vi "Measurement UI.vi"() -> ()   [LabVIEW 2023, in "Crosstalk_Class D Amplifier UI.lvlib"]
uses:
  Crosstalk_Class D Amplifier UI.lvlib
  shared/controls/digital output level units.ctl
  shared/ui/controls/view.ctl
  UI State.ctl
  <vilib>/Utility/miscctls.llb/LVBoundsTypeDef.ctl
  <vilib>/Utility/miscctls.llb/LVPoint32TypeDef.ctl
  <vilib>/Utility/miscctls.llb/LVPointTypeDef.ctl
  shared/ui/UI Helpers.lvlib
  shared/audio popup ui/Audio Popup UI.lvlib
  shared/controls/audio controls.lvlib
panel:
  in  "view legend":T1
  out "time domain":waveform(dbl)[](graph)
  out "frequency domain":T2(graph)
  out "meas table":string[][](table)
  in  "digital serial cfg file":string
  out "output power (W)":dbl[](array[numeric])
  out "crosstalk (dB)":dbl[](array[numeric])
  out "frequency (Hz)":dbl[](array[numeric])
  out "channel names":string[](array[string])
  in  "acq channel - interferer":string caption="Interferrer channel resource"
  in  "acq channel - victim":string caption="Victim channel resource"
  out "wfm_interferrer - data":dbl[](array[numeric])
  out "fft_interferrer - data":dbl[](array[numeric])
  in  "Configuration tab":enum32{"Protocol", "Measurement"}(tab)
  out "digital serial file name":string
  in  "configure digital serial":bool
  in  "master clock channel list":string caption="Master Clock Channel"
  in  "digital channel list":string caption="Digital Audio Channel"
  in  "Interferer channel resource":tag
  in  "Victim channel resource":tag
  in  "output level":dbl=-1.0 caption="Output level" format="%#_3f"
  in  "output level units":T3=enum."dBFS"
  in  "min settling cycles":u32 caption="Minimum settling cycles"
  in  "min settling time (s)":dbl=0.1 caption="Minimum settling time" format="%#_6ps"
  in  "min measurement cycles":u32 caption="Minimum measurement cycles"
  in  "min measurement time (s)":dbl=0.1 caption="Minimum measurement time" format="%#_6ps"
  in  "lowpass filter":T4(ring) caption="Lowpass filter"
  in  "highpass filter":enum32{"DC", "AC"}(ring) caption="Highpass filter"
  in  "load impedance":dbl=-1.0 caption="Load impedance" format="%#_6p Ohms"
  in  "digital audio interferer channel":i32 caption="Interferer channel"
  in  "output range (pk-pk)":dbl=15.0 caption="Output range" format="%.3p Vpk-pk"
  in  "signal frequency":dbl=1000.0 caption="Frequency" format="%#_6pHz"
  in  "acq sampling rate":dbl=51200.0 caption="Sample rate" format="%#.6pHz"
  in  "channel 0 offset":u32=1
  out "fft_victim - data":dbl[](array[numeric])
  out "fft - df":dbl
  out "fft - f0":dbl
  out "wfm_victim - data":dbl[](array[numeric])
  out "wfm - dt":dbl
  in  "acq channel":string="PXI1Slot4/ai0"
  in  "signal phase":dbl caption="phase"
  # "hidden controls - used to sync with MeasLink"
  # "hidden indicators"
  # "Digital Serial Settings"
  # "Harware Resource"
  # "Filters"
  # "Output"
  # "Acquisition"
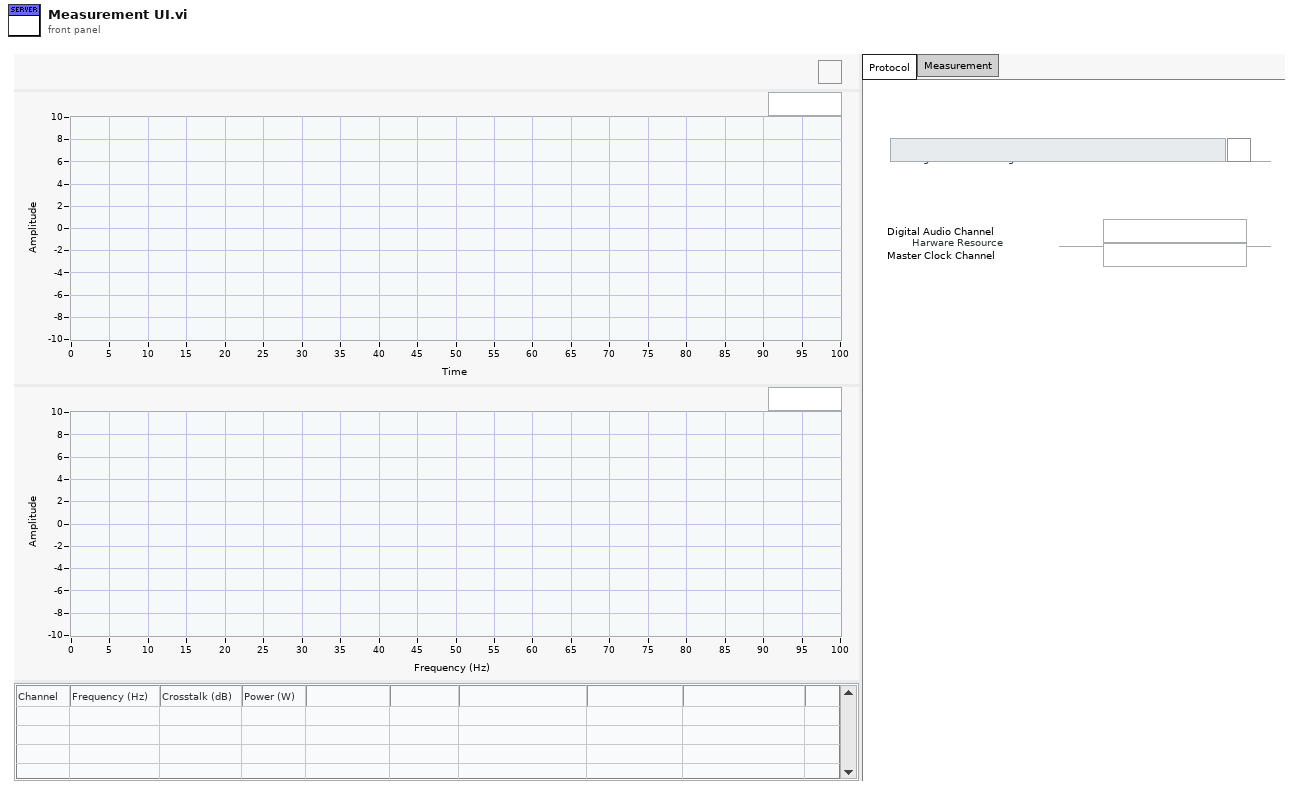
[diagram p1: front panel]
types:
  T1 = typedef "UI Helpers.lvlib/view.ctl" = bool
  T2 = cluster{"fft - f0":dbl, "fft - df":dbl, "fft_interferrer - data":dbl[]}[]
  T3 = typedef "audio controls.lvlib/digital output level units.ctl" = enum32{"% FS", "dBFS", "V"}
  T4 = enum32{"No filter", "AES17 20kHz", "AES17 40kHz"}
  T5 = typedef "Crosstalk_Class D Amplifier UI.lvlib/UI State.ctl" = cluster{"Graph Size":T6, "Legend Visible":bool, "Mouse Coords":T7, "PostUI event occurred":bool, "digital serial cfg file":path}
  T6 = typedef "LVBoundsTypeDef.ctl" = cluster{"Width":u32, "Height":u32}
  T7 = typedef "LVPoint32TypeDef.ctl" = cluster{"Horizontal":i32, "Vertical":i32}
  T8 = typedef "LVPointTypeDef.ctl" = cluster{"Horizontal":i16, "Vertical":i16}
  T9 = typedef "Audio Popup UI.lvlib/audio settings.ctl" = cluster{"digital serial file":string}
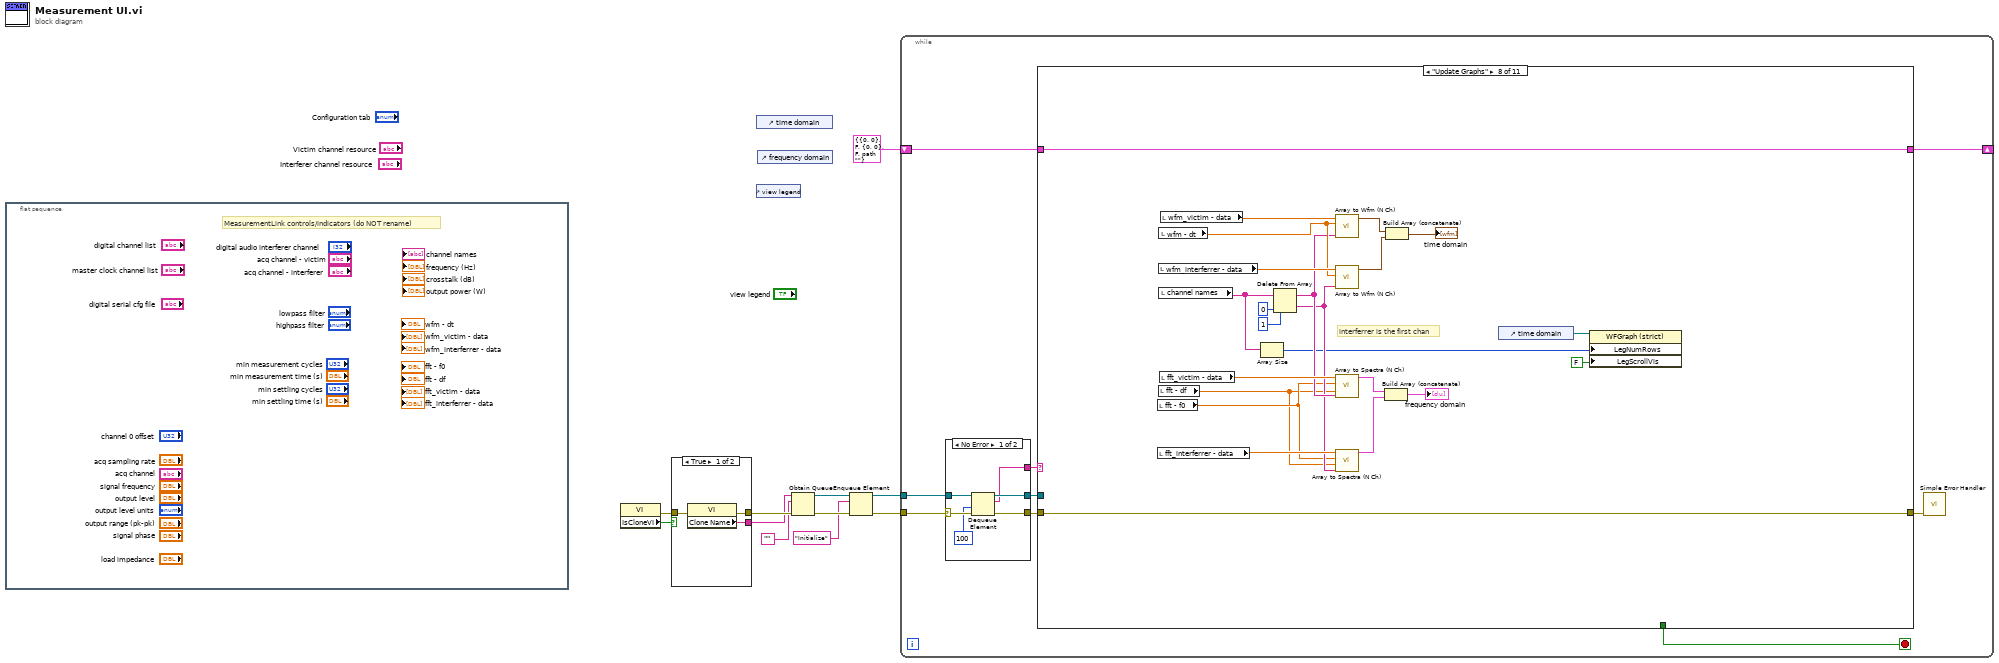
[diagram p0: block diagram]
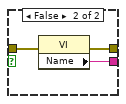
[diagram p2: hidden frame]
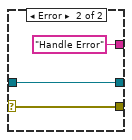
[diagram p3: hidden frame]
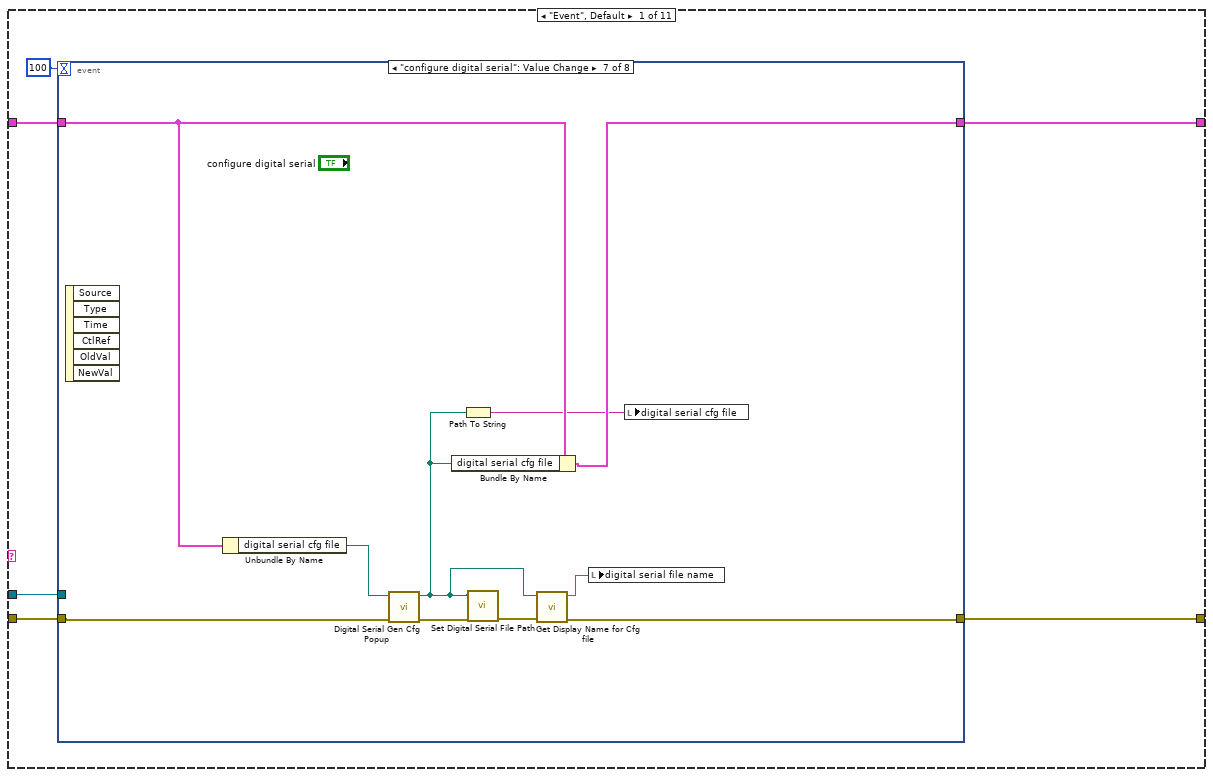
[diagram p4: hidden frame]
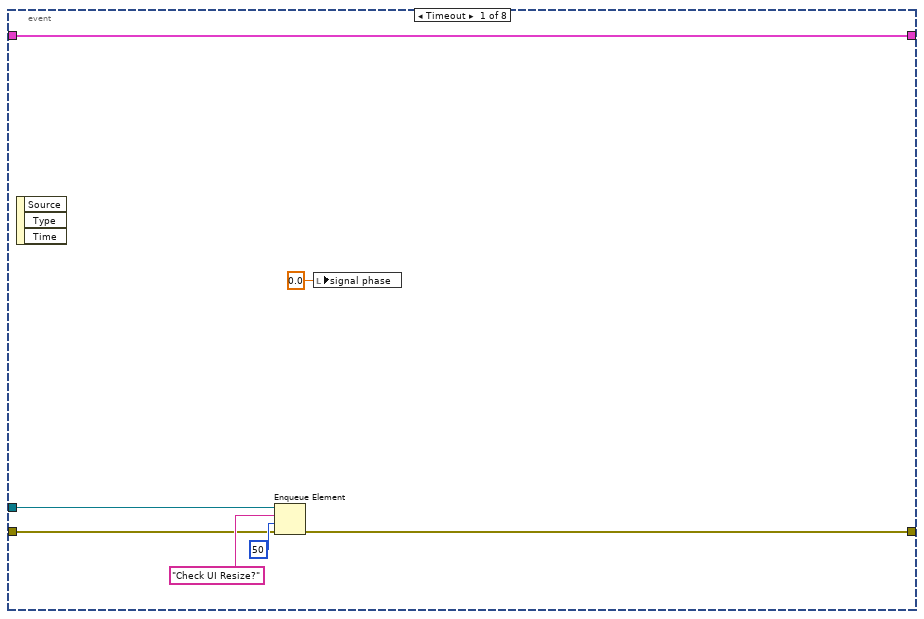
[diagram p5: hidden frame]
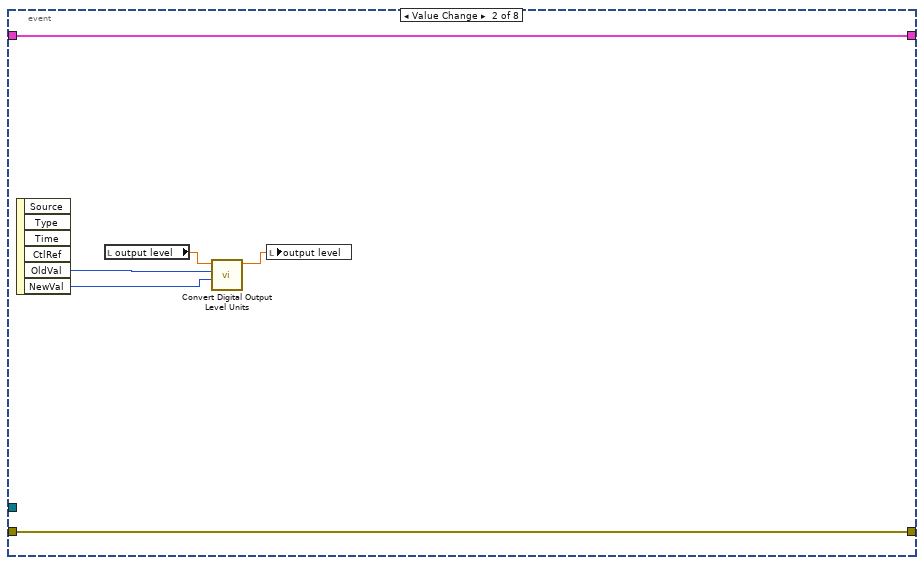
[diagram p6: hidden frame]
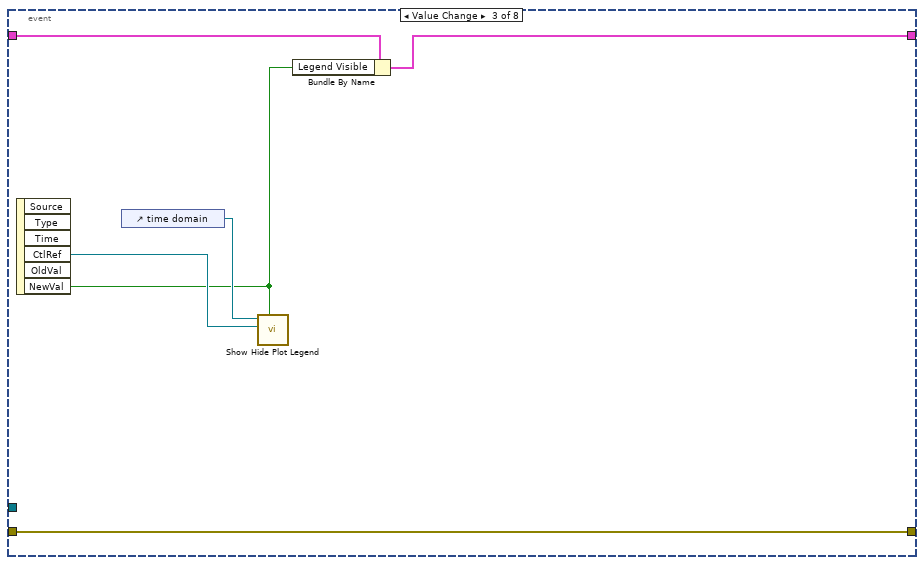
[diagram p7: hidden frame]
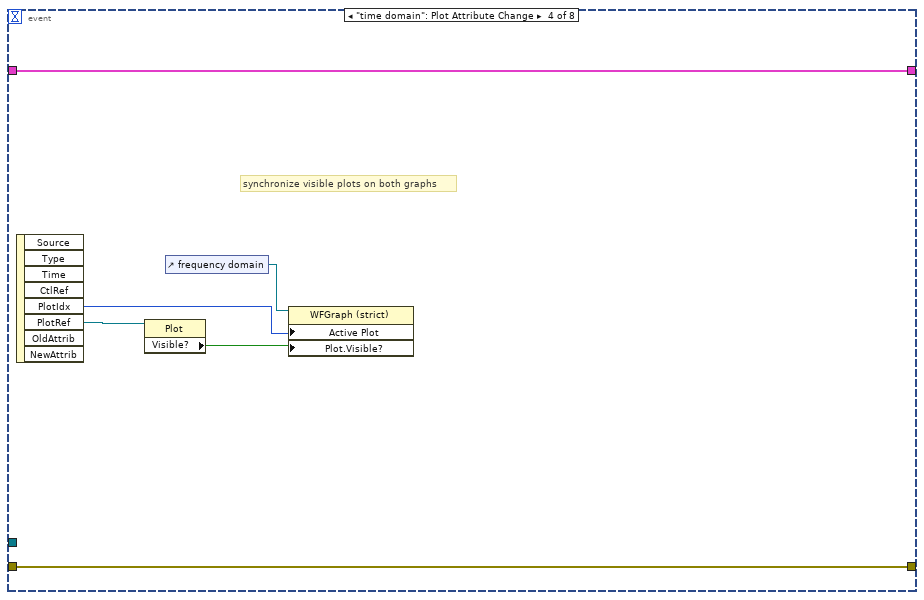
[diagram p8: hidden frame]
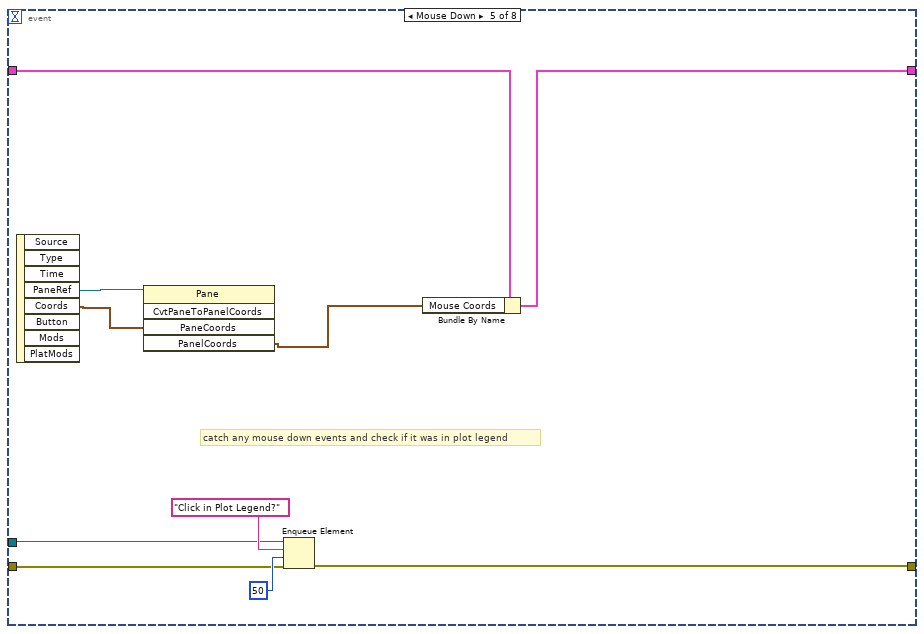
[diagram p9: hidden frame]
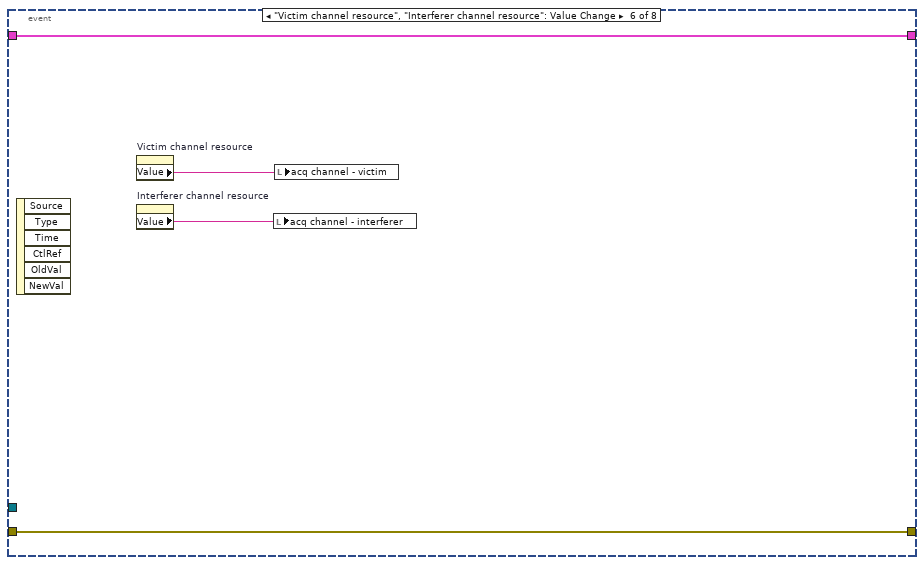
[diagram p10: hidden frame]
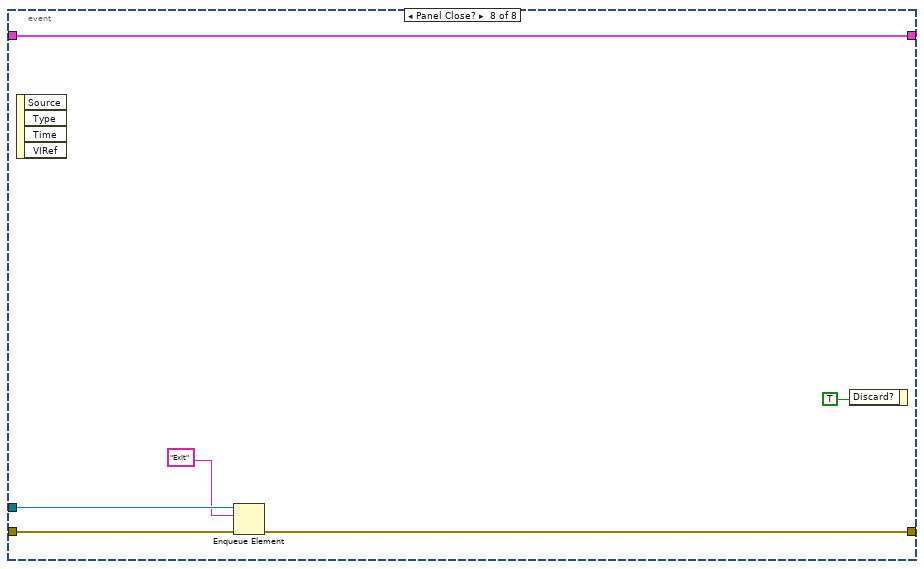
[diagram p11: hidden frame]
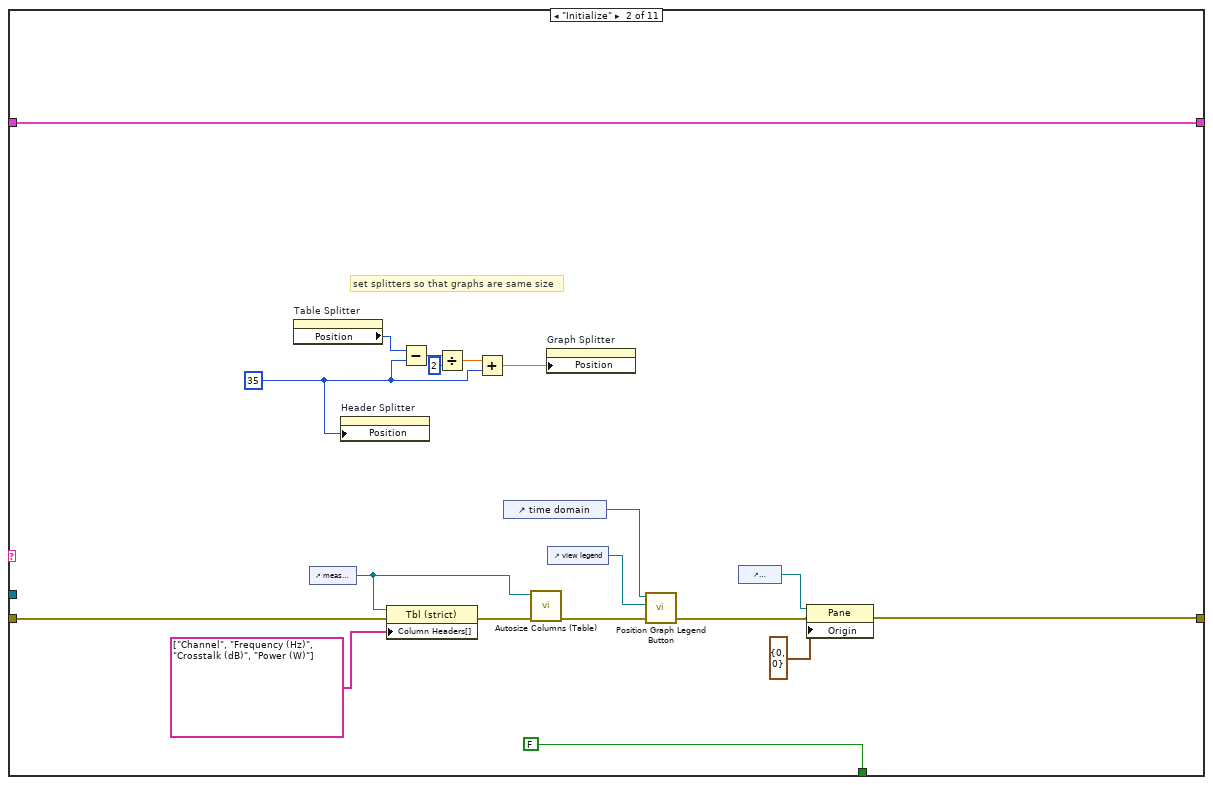
[diagram p12: hidden frame]
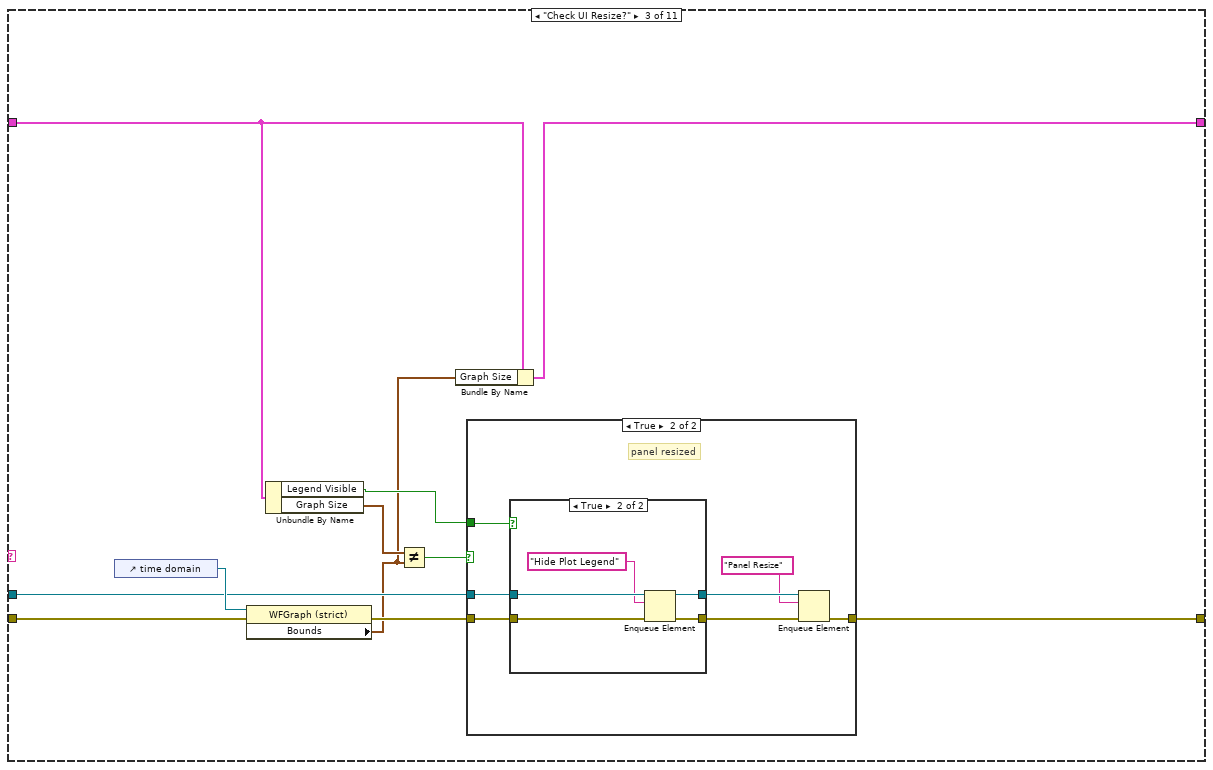
[diagram p13: hidden frame]
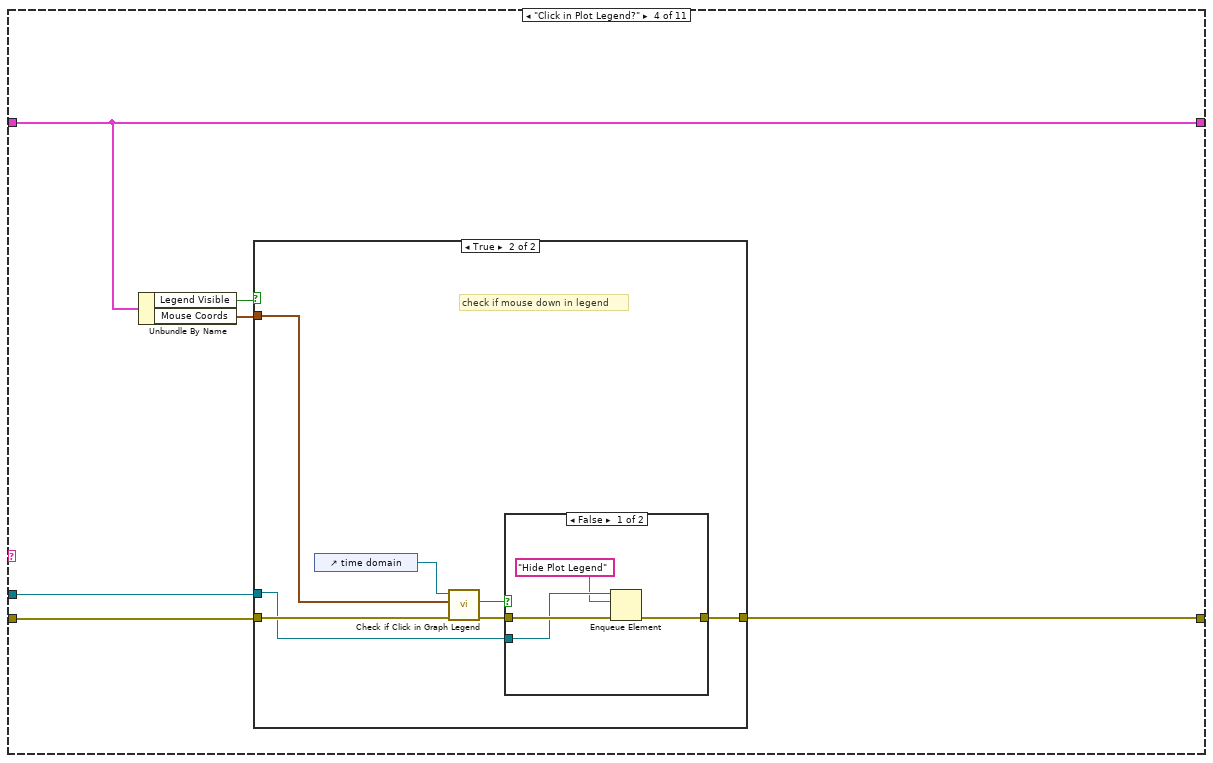
[diagram p16: hidden frame]
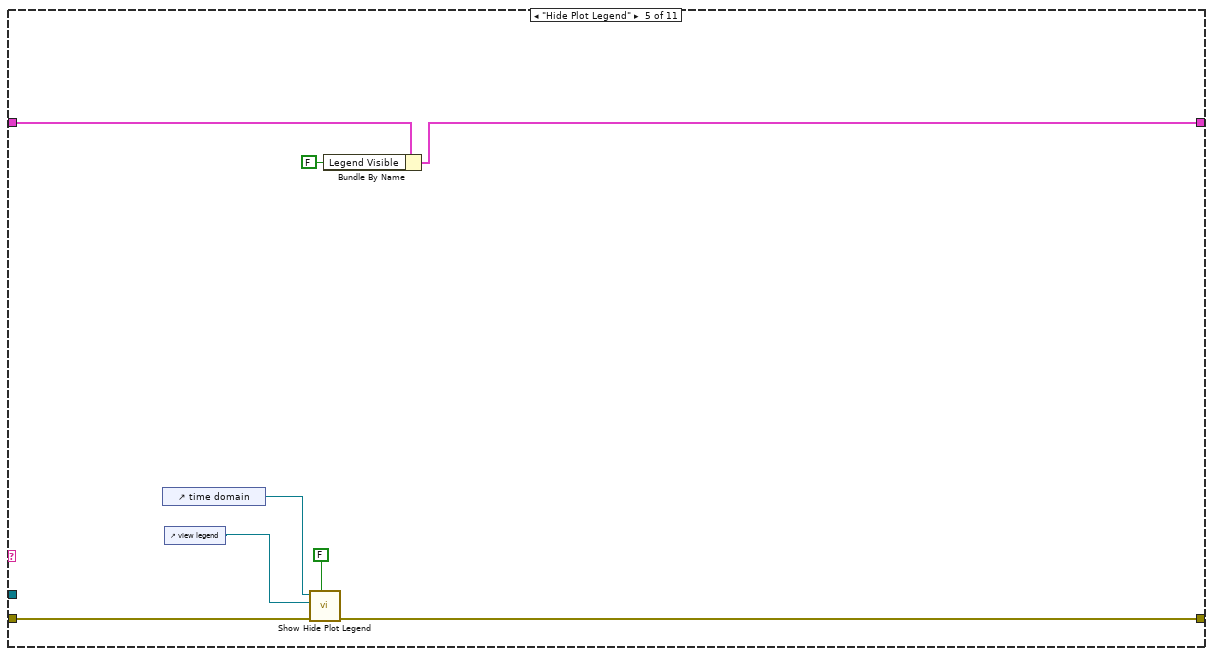
[diagram p19: hidden frame]
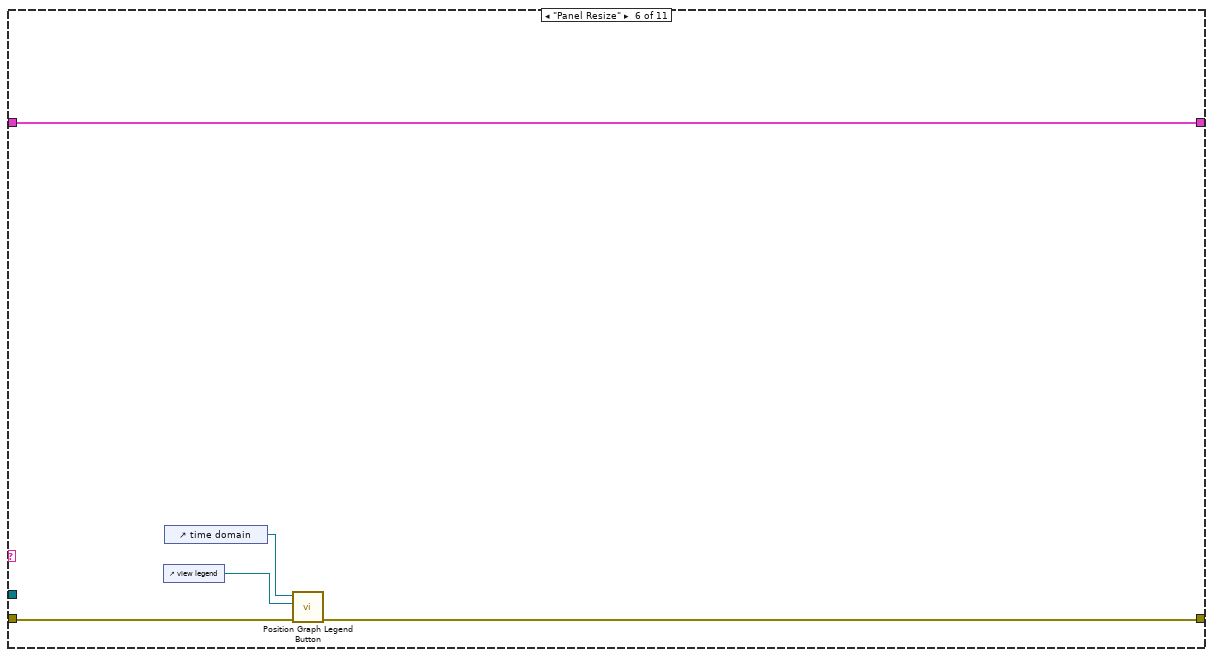
[diagram p20: hidden frame]
diagram:
  n1 = flat-sequence {
    frame #0 {
      # "MeasurementLink controls/indicators (do NOT rename)"
    }
  }
  n2 = property class="VI"() -> (error out=w2:errorcluster, "IsCloneVI"=w3:bool)  [unwired: 2 in, 1 out]
  n3 = case shown="True" w3 {
    tunnel: [w14 w17] -> w11
    tunnel: [w13 w16] -> w10
    tunnel: w2 -> [w12 w15]
    frame True {
      n4 = property class="VI"(error in=w12) -> (error out=w14:errorcluster, "Clone Name"=w13:string)  [unwired: 1 in, 1 out]
    }
    frame False {
      n5 = property class="VI"(error in=w15) -> (error out=w17:errorcluster, "Name"=w16:string)  [unwired: 1 in, 1 out]
    }
  }
  n6 = control-ref of="view legend"() -> ()  [unwired: 1 out]
  n7 = control-ref of="time domain"() -> ()  [unwired: 1 out]
  n8 = control-ref of="frequency domain"() -> ()  [unwired: 1 out]
  n9 = Obtain Queue(name (unnamed)=w10, element data type="", error in (no error)=w11) -> (queue out=w7:refnum<queue>, error out=w9:errorcluster)  [unwired: 2 in, 1 out]
  n10 = Enqueue Element(queue=w7, element="Initialize", error in (no error)=w9) -> (queue out=w6:refnum<queue>, error out=w8:errorcluster)  [unwired: 1 in, 1 out]
  n11 = while {
    tunnel: w6 -> [w24]
    shift-right: [w20] -> _
    shift-left: T5 {"Graph Size"={"Width"=0, "Height"=0}, "Legend Visible"=FALSE, "Mouse Coords"={"Horizontal"=0, "Vertical"=0}, "PostUI event occurred"=FALSE, "digital serial cfg file"=path ""} ("UI State") -> [w19]
    tunnel: w8 -> [w26]
    stop <- w21 stop-if-true
    n12 = case shown="No Error" w26 {
      selector: w26 -> [w32 w35]
      tunnel: [w31 w35] -> w25
      tunnel: w24 -> [w30 w34]
      tunnel: [w29 w34] -> w23
      tunnel: [w28 "Handle Error"] -> w22
      frame No Error {
        n13 = Dequeue Element(queue=w30, timeout in ms (-1)=100, error in (no error)=w32) -> (queue out=w29:refnum<queue>, element=w28:string, error out=w31:errorcluster)  [unwired: 1 out]
      }
      frame Error {
      }
    }
    n14 = case shown="\"Update Graphs\"" w22 {
      tunnel: w25 -> [w40 w113 w125 w146 w167 w171 w178 w227 w230 w265 w267]
      tunnel: w23 -> [w38 _ w117 w145 _ _ w179 _ _ w263 _]
      tunnel: [w41 w100 w116 w141 w166 w170 w173 w227 w231 w260 w267] -> w18
      tunnel: [_ FALSE _ _ _ _ _ _ _ TRUE _] -> w21
      tunnel: [w36 w97 w118 w142 w160 w172 w175 w229 w245 w258 w266] -> w20
      tunnel: w19 -> [w37 w97 w119 w142 w161 w172 w176 w229 w245 w258 w266]
      frame "Event", Default {
        n15 = event shown="[6] \"configure digital serial\": Value Change" {
          selector: _ -> [_ _ _ _ _ _ _ _]
          dyn-events: _ -> [_ _ _ _ _ _ _ _]
          timeout: 100 -> [_ _ _ _ _ _ _ _]
          tunnel: [w42 w49 w58 w66 w70 w77 w84 w94] -> w41
          tunnel: w40 -> [w44 w49 w58 w66 w72 w77 w87 w95]
          tunnel: w38 -> [w43 _ _ _ w71 _ _ w93]
          tunnel: w37 -> [w47 w50 w57 w65 w76 w78 w86 w91]
          tunnel: [w47 w50 w56 w65 w75 w78 w85 w91] -> w36
          event Timeout {
            n16 = event-data() -> ()  [unwired: 1 in, 3 out]
            n17 = Enqueue Element(queue=w43, element="Check UI Resize?", timeout in ms (-1)=50, error in (no error)=w44) -> (error out=w42:errorcluster)  [unwired: 2 out]
            n18 = local write "signal phase"(0.0 ("signal phase")) -> ()
          }
          event Value Change {
            n19 = event-data() -> ("OldVal"=w54:T3, "NewVal"=w53:T3)  [unwired: 1 in, 4 out]
            n20 = local read "output level"() -> (w51:dbl)
            n21 = call "Convert Digital Output Level Units.vi"("new output level units"=w53, "previous output level units"=w54, "previous output level"=w51) -> ("new output level"=w52:dbl)  [unwired: 8 in]
            n22 = local write "output level"(w52) -> ()
          }
          event Value Change {
            n23 = event-data() -> ("CtlRef"=w60:refnum<vi>, "NewVal"=w55:T1)  [unwired: 1 in, 4 out]
            n24 = control-ref of="time domain"() -> (w59:refnum<vi>)
            n25 = call "Show Hide Plot Legend.vi"("show"=w55, "view reference"=w60, "graph reference"=w59) -> ()  [unwired: 8 in, 1 out]
            n26 = Bundle By Name(cluster=w57, "Legend Visible"=w55) -> (w56:T5)
          }
          event "time domain": Plot Attribute Change {
            # "synchronize visible plots on both graphs"
            n27 = event-data() -> ("PlotIdx"=w62:i32, "PlotRef"=w63:refnum<vi>)  [unwired: 1 in, 6 out]
            n28 = property class="Plot"(reference=w63) -> ("Visible?"=w64:bool)  [unwired: 1 in, 2 out]
            n29 = control-ref of="frequency domain"() -> (w61:refnum<vi>)
            n30 = property on="Property Node" class="WFGraph (strict)"(reference=w61, "Active Plot"=w62, "Plot.Visible?"=w64) -> ()  [unwired: 1 in, 2 out]
          }
          event Mouse Down {
            # "catch any mouse down events and check if it was in plot legend"
            n31 = event-data() -> ("PaneRef"=w69:refnum<vi>, "Coords"=w68:T7)  [unwired: 1 in, 6 out]
            n32 = invoke class="Pane" method="CvtPaneToPanelCoords"(reference=w69, "PaneCoords"=w68) -> ("PanelCoords"=w67:T8)  [unwired: 3 in, 4 out]
            n33 = Enqueue Element(queue=w71, element="Click in Plot Legend?", timeout in ms (-1)=50, error in (no error)=w72) -> (error out=w70:errorcluster)  [unwired: 2 out]
            n34 = Bundle By Name(cluster=w76, "Mouse Coords"=w67) -> (w75:T5)
          }
          event "Victim channel resource", "Interferer channel resource": Value Change {
            n35 = event-data() -> ()  [unwired: 1 in, 6 out]
            n36 = property on="Victim channel resource" class="DAQmxName"() -> ("Value"=w80:string)  [unwired: 2 in, 2 out]
            n37 = property on="Interferer channel resource" class="DAQmxName"() -> ("Value"=w79:string)  [unwired: 2 in, 2 out]
            n38 = local write "acq channel - interferer"(w79) -> ()
            n39 = local write "acq channel - victim"(w80) -> ()
          }
          event "configure digital serial": Value Change {
            n40 = event-data() -> ()  [unwired: 1 in, 6 out]
            n41 = Unbundle By Name(w86) -> ("digital serial cfg file"=w90:path)
            n42 = call "Digital Serial Gen Cfg Popup.vi"("error in (no error)"=w87, "config file in"=w90) -> ("error out"=w89:errorcluster, "config file out"=w83:path)  [unwired: 7 in, 1 out]
            n43 = Bundle By Name(cluster=w86, "digital serial cfg file"=w83) -> (w85:T5)
            n44 = Path To String(path=w83) -> (string=w82:string)
            n45 = call "Set Digital Serial File Path.vi"("error in (no error)"=w89, "digital serial file"=w83) -> ("error out"=w88:errorcluster)  [unwired: 9 in]
            n46 = call "Get Display Name for Cfg file.vi"("error in (no error)"=w88, "file path"=w83) -> ("error out"=w84:errorcluster, "display string"=w81:string)  [unwired: 8 in]
            n47 = local write "digital serial file name"(w81) -> ()
            n48 = local write "digital serial cfg file"(w82) -> ()
          }
          event Panel Close? {
            n49 = event-data() -> ()  [unwired: 1 in, 4 out]
            n50 = Enqueue Element(queue=w93, element="Exit", error in (no error)=w95) -> (error out=w94:errorcluster)  [unwired: 1 in, 2 out]
            n51 = event-data("Discard?"=TRUE) -> ()  [unwired: 1 in, 1 out]
          }
        }
      }
      frame "Initialize" {
        w102 = 35 ("Splitter Position")
        # "set splitters so that graphs are same size"
        n52 = property on="Table Splitter" class="Splitter"() -> ("Position"=w109:i32)  [unwired: 2 in, 2 out]
        n53 = control-ref of="meas table"() -> (w112:refnum<vi>)
        n54 = property on="Header Splitter" class="Splitter"("Position"=w102) -> ()  [unwired: 2 in, 2 out]
        n55 = property class="Tbl (strict)"(reference=w112, error in=w113, "Column Headers[]"=string[] ["Channel", "Frequency (Hz)", "Crosstalk (dB)", "Power (W)"] ("Column Header Strings[]")) -> (error out=w111:errorcluster)  [unwired: 1 out]
        n56 = Subtract(x=w109, y=w102) -> (x-y=w108:i32)
        n57 = Divide(x=w108, y=2) -> (x/y=w106:dbl)
        n58 = Add(x=w106, y=w102) -> (x+y=w105:dbl)
        n59 = control-ref of="time domain"() -> (w103:refnum<vi>)
        n60 = call "Autosize Columns (Table).vi"("error in (no error)"=w111, "table"=w112) -> ("error out"=w101:errorcluster)  [unwired: 9 in]
        n61 = property on="Graph Splitter" class="Splitter"("Position"=w105) -> ()  [unwired: 2 in, 2 out]
        n62 = control-ref of="view legend"() -> (w104:refnum<vi>)
        n63 = call "Position Graph Legend Button.vi"("view legend"=w104, "graph"=w103) -> ()  [unwired: 9 in, 1 out]
        n64 = control-ref of="Configuration"() -> (w99:refnum<vi>)
        n65 = property class="Pane"(reference=w99, error in=w101, "Origin"=T8 {"Horizontal"=0, "Vertical"=0}) -> (error out=w100:errorcluster)  [unwired: 1 out]
      }
      frame "Check UI Resize?" {
        n66 = control-ref of="time domain"() -> (w123:refnum<vi>)
        n67 = property on="Property Node" class="WFGraph (strict)"(reference=w123, error in=w125) -> (error out=w124:errorcluster, "Bounds"=w115:T6)  [unwired: 1 out]
        n68 = Unbundle By Name(w119) -> ("Legend Visible"=w121:bool, "Graph Size"=w120:T6)
        n69 = Not Equal?(x=w120, y=w115) -> (x != y?=w122:bool)
        n70 = Bundle By Name(cluster=w119, "Graph Size"=w115) -> (w118:T5)
        n71 = case shown="True" w122 {
          tunnel: w124 -> [w126 w133]
          tunnel: [w126 w128] -> w116
          tunnel: w121 -> [_ w131]
          tunnel: w117 -> [_ w132]
          frame False {
            # "no resize"
          }
          frame True {
            # "panel resized"
            n72 = case shown="True" w131 {
              tunnel: w133 -> [w135 w140]
              tunnel: [w135 w139] -> w130
              tunnel: w132 -> [w134 w138]
              tunnel: [w134 w136] -> w129
              frame False {
              }
              frame True {
                n73 = Enqueue Element(queue=w138, element="Hide Plot Legend", error in (no error)=w140) -> (queue out=w136:refnum<queue>, error out=w139:errorcluster)  [unwired: 1 in, 1 out]
              }
            }
            n74 = Enqueue Element(queue=w129, element="Panel Resize", error in (no error)=w130) -> (error out=w128:errorcluster)  [unwired: 1 in, 2 out]
          }
        }
      }
      frame "Click in Plot Legend?" {
        n75 = Unbundle By Name(w142) -> ("Legend Visible"=w143:bool, "Mouse Coords"=w144:T7)
        n76 = case shown="True" w143 {
          tunnel: w144 -> [_ w153]
          tunnel: w145 -> [_ w150]
          tunnel: w146 -> [w147 w154]
          tunnel: [w147 w149] -> w141
          frame False {
            # "legend not visible; do nothing"
          }
          frame True {
            # "check if mouse down in legend"
            n77 = control-ref of="time domain"() -> (w148:refnum<vi>)
            n78 = call "Check if Click in Graph Legend.vi"("error in (no error)"=w154, "Mouse Coords"=w153, "WaveformGraph"=w148) -> ("error out"=w151:errorcluster, "click in legend?"=w152:bool)  [unwired: 7 in]
            n79 = case shown="False" w152 {
              tunnel: w151 -> [w158 w159]
              tunnel: w150 -> [w157 _]
              tunnel: [w156 w159] -> w149
              frame False {
                n80 = Enqueue Element(queue=w157, element="Hide Plot Legend", error in (no error)=w158) -> (error out=w156:errorcluster)  [unwired: 1 in, 2 out]
              }
              frame True {
                # "inside legend; do nothing"
              }
            }
          }
        }
      }
      frame "Hide Plot Legend" {
        n81 = control-ref of="time domain"() -> (w165:refnum<vi>)
        n82 = control-ref of="view legend"() -> (w163:refnum<vi>)
        n83 = call "Show Hide Plot Legend.vi"("show"=FALSE, "error in (no error)"=w167, "view reference"=w163, "graph reference"=w165) -> ("error out"=w166:errorcluster)  [unwired: 7 in]
        n84 = Bundle By Name(cluster=w161, "Legend Visible"=FALSE ("legend visible")) -> (w160:T5)
      }
      frame "Panel Resize" {
        n85 = control-ref of="view legend"() -> (w168:refnum<vi>)
        n86 = control-ref of="time domain"() -> (w169:refnum<vi>)
        n87 = call "Position Graph Legend Button.vi"("error in (no error)"=w171, "view legend"=w168, "graph"=w169) -> ("error out"=w170:errorcluster)  [unwired: 8 in]
      }
      frame "Post UI Update" {
        # "This case will be triggered, after framework updates the User interface with result values."
        n88 = Unbundle By Name(w176) -> ("PostUI event occurred"=w177:bool)
        n89 = for {
          tunnel: w179 -> [w204]
          shift-right: [w203] -> w174
          shift-left: w178 -> [w205]
          tunnel: string[] ["Update Table", "Update Graphs"] -> [w202] mode=indexing
          n90 = Enqueue Element(queue=w204, element=w202, timeout in ms (-1)=50, error in (no error)=w205) -> (error out=w203:errorcluster)  [unwired: 2 out]
        }
        n91 = case shown="False" w177 {
          tunnel: w176 -> [w191 w201]
          tunnel: [w190 w201] -> w175
          tunnel: w174 -> [w186 w200]
          tunnel: [w185 w200] -> w173
          frame False {
            # "do this on first PostUI Event (happens when panel loads)"
            # "Initialize the DAQmx channel control"
            n92 = local read "digital serial cfg file"() -> (w184:string)
            n93 = local read "acq channel - interferer"() -> (w193:string)
            n94 = local read "acq channel - victim"() -> (w192:string)
            n95 = Empty String/Path?(string/path=w184) -> (empty?=w188:bool)
            n96 = case shown="True" w188 {
              tunnel: w186 -> [w195 w199]
              tunnel: [w195 w197] -> w187
              tunnel: w184 -> [w194 _]
              tunnel: [w194 w196] -> w181
              frame False {
              }
              frame True {
                n97 = call "Get Audio Settings.vi"("error in (no error)"=w199) -> ("error out"=w197:errorcluster, "audio settings"=w198:T9)  [unwired: 9 in]
                n98 = Unbundle By Name(w198) -> ("digital serial file"=w196:string)
              }
            }
            n99 = property on="Victim channel resource" class="DAQmxName"("Value"=w192) -> ()  [unwired: 2 in, 2 out]
            n100 = property on="Interferer channel resource" class="DAQmxName"("Value"=w193) -> ()  [unwired: 2 in, 2 out]
            n101 = String To Path(string=w181) -> (path=w182:path)
            n102 = local write "digital serial cfg file"(w181) -> ()
            n103 = call "Get Display Name for Cfg file.vi"("error in (no error)"=w187, "file path"=w182) -> ("error out"=w185:errorcluster, "display string"=→"digital serial file name":string)  [unwired: 8 in]
            n104 = Bundle By Name(cluster=w191, "PostUI event occurred"=TRUE, "digital serial cfg file"=w182) -> (w190:T5)
          }
          frame True {
          }
        }
      }
      frame "Update Graphs" {
        # "interferrer is the first chan"
        n105 = local read "fft - f0"() -> (w208:dbl)
        n106 = local read "fft_interferrer - data"() -> (w217:dbl[])
        n107 = local read "wfm_interferrer - data"() -> (w224:dbl[])
        n108 = local read "fft - df"() -> (w207:dbl)
        n109 = local read "wfm - dt"() -> (w223:dbl)
        n110 = local read "channel names"() -> (w212:string[])
        n111 = local read "fft_victim - data"() -> (w218:dbl[])
        n112 = local read "wfm_victim - data"() -> (w225:dbl[])
        n113 = Array Size(array=w212) -> (size(s)=w211:i32)
        n114 = Delete From Array(array=w212, length=1, index=0) -> (deleted portion=w215:string[], array with subset deleted=w216:string[])
        n115 = call "Array to Wfm (N Ch).vi"("channel names"=w216, "dt"=w223, "array"=w225) -> ("waveforms"=w226:waveform(dbl)[])  [unwired: 8 in]
        n116 = call "Array to Wfm (N Ch).vi"("channel names"=w215, "dt"=w223, "array"=w224) -> ("waveforms"=w222:waveform(dbl)[])  [unwired: 8 in]
        n117 = call "Array to Spectra (N Ch).vi"("channel names"=w216, "df"=w207, "f0"=w208, "data"=w218) -> ("spectra"=w210:cluster{"f0":dbl, "df":dbl, "data":dbl[]}[])  [unwired: 7 in]
        n118 = call "Array to Spectra (N Ch).vi"("channel names"=w215, "df"=w207, "f0"=w208, "data"=w217) -> ("spectra"=w209:cluster{"f0":dbl, "df":dbl, "data":dbl[]}[])  [unwired: 7 in]
        n119 = Build Array (concatenate)(w210, w209) -> (→"frequency domain":cluster{"f0":dbl, "df":dbl, "data":dbl[]}[])
        n120 = Build Array (concatenate)(w226, w222) -> (→"time domain":waveform(dbl)[])
        n121 = control-ref of="time domain"() -> (w213:refnum<vi>)
        n122 = property class="WFGraph (strict)"(reference=w213, "LegNumRows"=w211, "LegScrollVis"=FALSE ("Legend:Scrollbar Visible")) -> ()  [unwired: 1 in, 2 out]
      }
      frame "Update Table" {
        n123 = local read "output power (W)"() -> (w237:dbl[])
        n124 = local read "channel names"() -> (w244:string[])
        n125 = local read "crosstalk (dB)"() -> (w238:dbl[])
        n126 = local read "frequency (Hz)"() -> (w241:dbl[])
        n127 = call "Format Channel Names - Crosstalk.vi"("names in"=w244) -> ("names out"=w243:string[])  [unwired: 10 in]
        n128 = for {
          tunnel: [w257] -> w242 mode=indexing
          tunnel: w241 -> [w256] mode=indexing
          tunnel: "%5.3f" ("initial string") -> [w255]
          n129 = Format Into String(format string=w255, w256) -> (resulting string=w257:string)  [unwired: 2 in, 1 out]
        }
        n130 = for {
          tunnel: [w254] -> w240 mode=indexing
          tunnel: "%5.1f" ("initial string") -> [w253]
          tunnel: w238 -> [w252] mode=indexing
          n131 = Format Into String(format string=w253, w252) -> (resulting string=w254:string)  [unwired: 2 in, 1 out]
        }
        n132 = for {
          tunnel: [w251] -> w239 mode=indexing
          tunnel: "%.3f" ("initial string") -> [w250]
          tunnel: w237 -> [w249] mode=indexing
          n133 = Format Into String(format string=w250, w249) -> (resulting string=w251:string)  [unwired: 2 in, 1 out]
        }
        n134 = Build Array(w243, w242, w240, w239) -> (w236:string[][])
        n135 = Transpose 2D Array(2D array=w236) -> (transposed array=w235:string[][])
        "meas table" <- w235
        n136 = flat-sequence {
          tunnel: w230 -> [w248]
          tunnel: [w247] -> w231
          tunnel: w235 -> [_]
          frame #0 {
            n137 = control-ref of="meas table"() -> (w246:refnum<vi>)
            n138 = call "Autosize Columns (Table).vi"("error in (no error)"=w248, "table"=w246) -> ("error out"=w247:errorcluster)  [unwired: 9 in]
          }
        }
      }
      frame "Exit" {
        # "This case is triggered to close the User Interface from framework"
        n139 = Flush Queue(queue=w263, error in (no error)=w265) -> (queue out=w262:refnum<queue>, error out=w261:errorcluster)  [unwired: 1 out]
        n140 = Release Queue(queue=w262, force destroy? (F)=TRUE, error in (no error)=w261) -> (error out=w260:errorcluster)  [unwired: 2 out]
      }
      frame "Handle Error" {
      }
    }
    n141 = call <vilib>:"Simple Error Handler.vi"("error in (no error)"=w18) -> ()  [unwired: 4 in, 5 out]
  }
